vi "GET_ERROR.vi"(7 "uLPtr":u32[](array[numeric]), 11 "error in (no error)":errorcluster) -> (4 "function return":string, 8 "uLPtr":u32[](array[numeric]), 15 "error out":errorcluster)   [LabVIEW 2017, in "ZBOX_IS.lvlib"]
uses:
  ZBOX_IS.lvlib
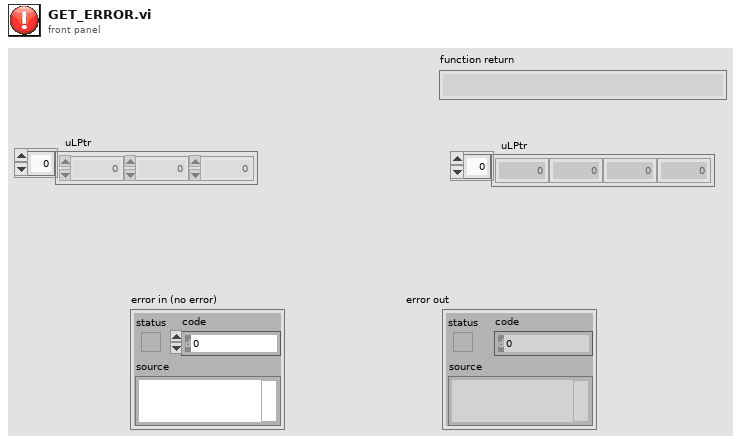
[diagram p1: front panel]
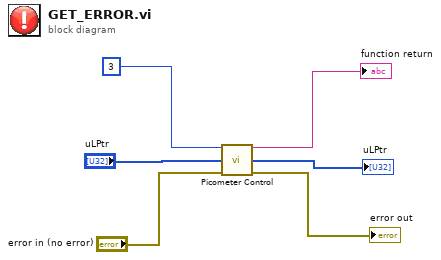
[diagram p0: block diagram]
diagram:
  n1 = call "Picometer Control.vi"("Cmd"=u8 3, "uLPtr"="uLPtr", "error in (no error)"="error in (no error)") -> ("function return"=→"function return":string, "uLPtr"=→"uLPtr":u32[], "error out"=→"error out":errorcluster)  [unwired: 8 in, 2 out]
